vi "InsetRect.vi"(8 "错误输入":errorcluster, 9 "dv":i16=1, 10 "dh":i16=1, 11 "rect":T1 caption="矩形") -> (0 "错误输出":errorcluster, 3 "inset rect":T1 caption="内缩矩形")   [LabVIEW 2012, in "Picture Box Tools.lvlib" / "Rect Tools.lvlib"]
uses:
  Rect Tools.lvlib
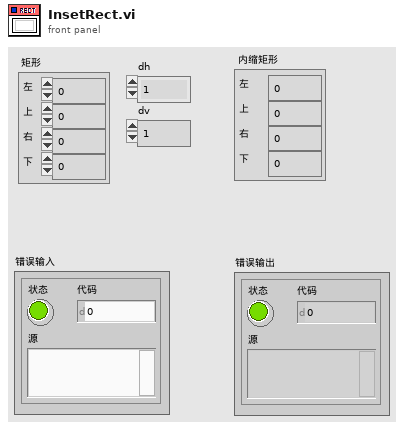
[diagram p1: front panel]
types:
  T1 = cluster{"left":i16, "top":i16, "right":i16, "bottom":i16}
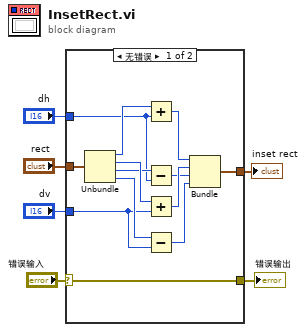
[diagram p0: block diagram]
diagram:
  n1 = case shown="无错误" "错误输入" {
    selector: "错误输入" -> [w11 w21]
    tunnel: [w11 w21] -> w5
    tunnel: "rect" -> [w10 w20]
    tunnel: [w9 w20] -> w3
    tunnel: "dv" -> [w8 _]
    tunnel: "dh" -> [w7 _]
    frame No Error {
      n2 = Unbundle(w10) -> ("left"=w19:i16, "top"=w17:i16, "right"=w15:i16, "bottom"=w13:i16)
      n3 = Add(x=w19, y=w7) -> (x+y=w18:i16)
      n4 = Subtract(x=w15, y=w7) -> (x-y=w14:i16)
      n5 = Add(x=w17, y=w8) -> (x+y=w16:i16)
      n6 = Subtract(x=w13, y=w8) -> (x-y=w12:i16)
      n7 = Bundle(w18, w16, w14, w12) -> (w9:cluster{i16, i16, i16, i16})  [unwired: 1 in]
    }
    frame Error {
    }
  }
  "错误输出" <- w5
  "inset rect" <- w3
